vi "AutoHide Windows Taskbar.vi"(4 "error in (no error)":errorcluster, 7 "Operation":u8(ring) items=["AutoHide"=1, "AlwaysOnTop"=2]) -> (0 "error out":errorcluster)   [LabVIEW 2016]
doc: "The AutoHide Windows Taskbar VI will programmatically show or autohide the Windows Taskbar. This can be useful if you need to use the full screen of the primary monitor and not allow the user access to the Start Menu with the mouse. Press <Ctrl-Esc> to show the Start Menu.\n\nThe VI calls the Windows API and uses the SHAppBarMessage function."
uses:
  shell32.dll
  user32.dll
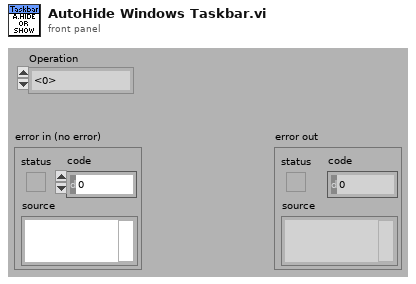
[diagram p1: front panel]
types:
  T1 = cluster{"cbSize":u32, "hWnd":i32, "uCallbakMessage":u32, "uEdge":u32, "rc":cluster{"left":i32, "top":i32, "right":i32, "bottom":i32}, "lParam":u8}
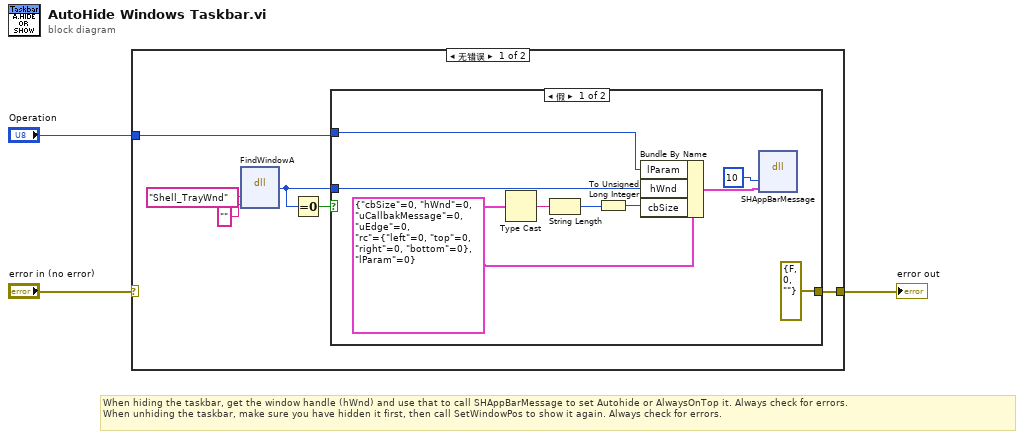
[diagram p0: block diagram]
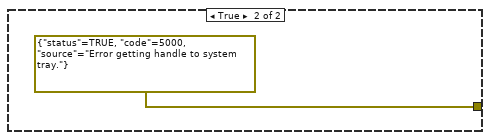
[diagram p2: hidden frame]
diagram:
  # "When hiding the taskbar, get the window handle (hWnd) and use that to call SHAppBarMessage to set Autohide or AlwaysOnTop it. Always check for errors.\nWhen unhiding the taskbar, make sure you have hidden it first, then call SetWindowPos to show it again. Always check for errors."
  n1 = case shown="无错误" "error in (no error)" {
    selector: "error in (no error)" -> [_ w20]
    tunnel: [w9 w20] -> w3
    tunnel: "Operation" -> [w4 _]
    frame No Error {
      n2 = dll-call lib="USER32.DLL" fn="FindWindowA"("lpClassName"="Shell_TrayWnd", "lpWindowName"="") -> ("hWnd"=w5:i32)  [unwired: 5 in, 2 out]
      n3 = Equal To 0?(x=w5) -> (x = 0?=w6:bool)
      n4 = case shown="假" w6 {
        tunnel: w5 -> [w14 _]
        tunnel: [errorcluster {"status"=FALSE, "code"=0, "source"=""} ("error out") errorcluster {"status"=TRUE, "code"=5000, "source"="Error getting handle to system tray."} ("error out")] -> w9
        tunnel: w4 -> [w11 _]
        frame False {
          w17 = T1 {"cbSize"=0, "hWnd"=0, "uCallbakMessage"=0, "uEdge"=0, "rc"={"left"=0, "top"=0, "right"=0, "bottom"=0}, "lParam"=0}
          n5 = Type Cast(x=w17) -> (*(type *) &x=w18:string)  [unwired: 1 in]
          n6 = String Length(string=w18) -> (length=w16:i32)
          n7 = To Unsigned Long Integer(number=w16) -> (unsigned 32bit integer=w15:u32)
          n8 = Bundle By Name(cluster=w17, "lParam"=w11, "hWnd"=w14, "cbSize"=w15) -> (w12:T1)
          n9 = dll-call lib="shell32.dll" fn="SHAppBarMessage"("dwMessage"=u32 10, "pData"=w12) -> ()  [unwired: 6 in, 2 out]
        }
        frame True {
        }
      }
    }
    frame Error {
      # "Previous Error. Pass it through."
    }
  }
  "error out" <- w3
